vi "Total induced velocity at point P.vi"(1 "U_inf":sgl[](array[numeric])=[1.0, 0.0, 0.0], 2 "P":sgl[](array[numeric])=[-1.0, 0.0, 0.0], 3 "Triangle panels":T1[](array[typedef])) -> (0 "(U, V, W) at P":sgl[](array[numeric])=[0.8764689, 4.19611e-11, 8.890311e-11])   [LabVIEW 2017]
uses:
  ctls/Triangle panel.ctl
  Biot-Savart induced velocity.vi
panel:
  # "PN 22/10/17"
  # "Vertices"
  # "Edges"
  # "Unit normal"
  # "Control point"
  # "Edge\nlinks \n(tri index)"
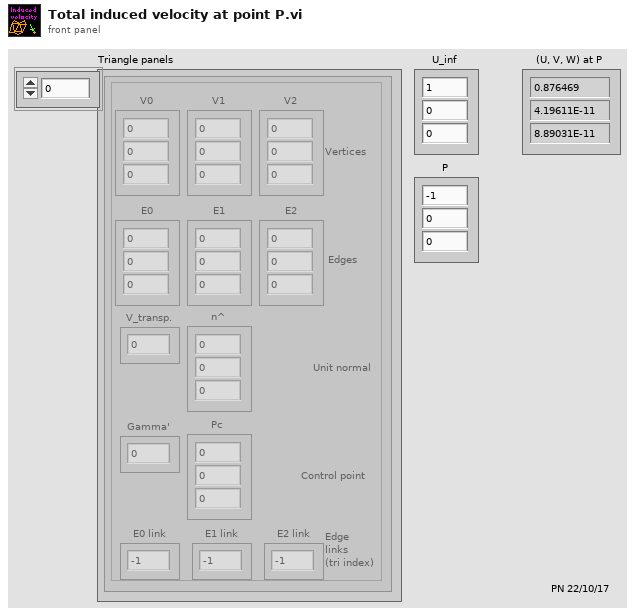
[diagram p1: front panel]
types:
  T1 = typedef "Triangle panel.ctl" = cluster{"V0":sgl[], "V1":sgl[], "V2":sgl[], "E0":sgl[], "E1":sgl[], "E2":sgl[], "n^":sgl[], "Pc":sgl[], "Gamma'":sgl, "V_transp.":sgl, "E0 link":i32, "E1 link":i32, "E2 link":i32}
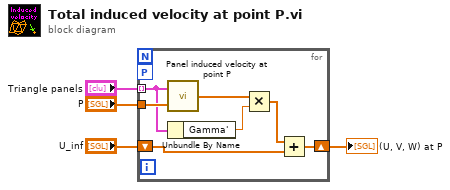
[diagram p0: block diagram]
diagram:
  n1 = for {
    tunnel: "P" -> [w11]
    tunnel: "Triangle panels" -> [w10] mode=indexing
    workers-P: _ -> [_]
    shift-right: [w7] -> w1
    shift-left: "U_inf" -> [w5]
    n2 = call "Panel induced velocity at point P.vi"("P"=w11, "Triangle panel"=w10) -> ("U / G'"=w8:sgl[])
    n3 = Unbundle By Name(w10) -> ("Gamma'"=w9:sgl)
    n4 = Multiply(x=w8, y=w9) -> (x*y=w6:sgl[])
    n5 = Add(x=w6, y=w5) -> (x+y=w7:sgl[])
  }
  "(U, V, W) at P" <- w1
